vi "uA_daq_switch_external_internal_pw_source.vi"(8 "error in":errorcluster, 10 "USB DAQ":tag="Dev4", 11 "Ex/Int PW":T1(ring)) -> (0 "error out":errorcluster)   [LabVIEW 2017]
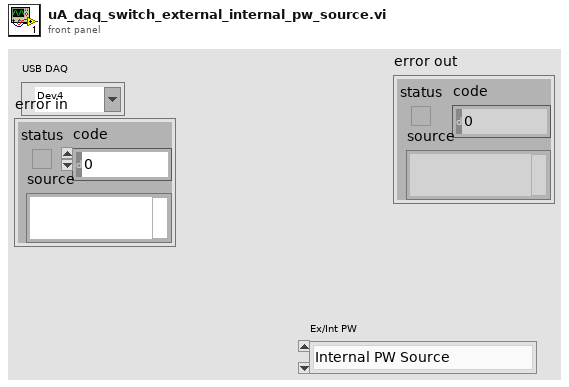
[diagram p1: front panel]
types:
  T1 = enum16{"Internal PW Source", "External PW Source"}
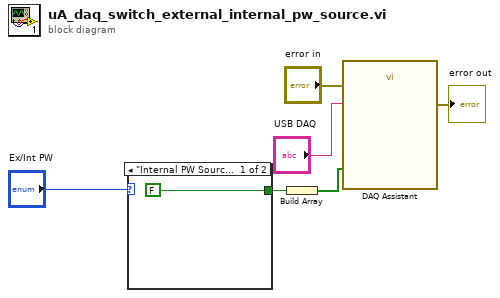
[diagram p0: block diagram]
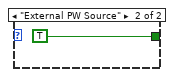
[diagram p2: hidden frame]
diagram:
  n1 = case shown="\"Internal PW Source\", Default" "Ex/Int PW" {
    tunnel: [FALSE TRUE] -> w5
    frame "Internal PW Source", Default {
    }
    frame "External PW Source" {
    }
  }
  n2 = Build Array(w5) -> (w4:bool[])
  n3 = call "DAQ Assistant"("data"=w4, "error in"="error in", "device name"="USB DAQ") -> ("error out"=→"error out":errorcluster)  [unwired: 15 in, 1 out]
